vi "Rx Inline Wait.vi"(8 "error in (no error)":errorcluster, 11 "Framework in":refnum<class "Framework.lvclass">) -> (0 "error out":errorcluster, 3 "Framework out":refnum<class "Framework.lvclass">)   [LabVIEW 2021, in "DSF Core.lvlib" / "Framework.lvclass"]
uses:
  Framework.lvclass
  Framework.lvclass/Framework.ctl
  Plugin/Plugin.lvclass
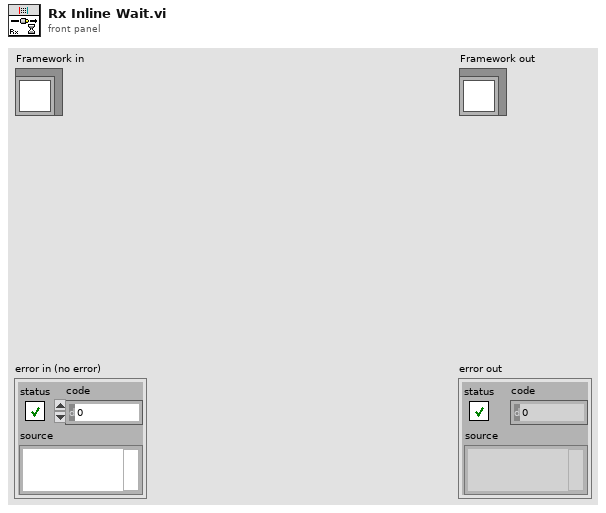
[diagram p1: front panel]
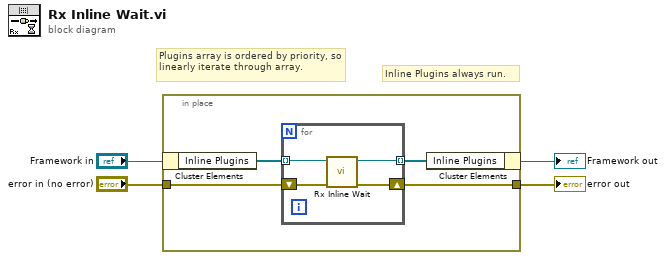
[diagram p0: block diagram]
diagram:
  # "Inline Plugins always run."
  # "Plugins array is ordered by priority, so linearly iterate through array."
  n1 = in-place {
    in-place-border: "error in (no error)" -> [w8]
    in-place-border: [w7] -> w3
    n2 = in-place-cluster #1("Framework in") -> ("Inline Plugins"=w6:refnum<class "Plugin.lvclass">[])
    n3 = for {
      tunnel: w6 -> [w9] mode=indexing
      tunnel: [w12] -> w5 mode=indexing
      shift-right: [w11] -> w7
      shift-left: w8 -> [w10]
      n4 = call "Rx Inline Wait.vi"("error in (no error)"=w10, "Plugin in"=w9) -> ("error out"=w11:errorcluster, "Plugin out"=w12:refnum<class "Plugin.lvclass">)  [unwired: 8 in]
    }
    n5 = in-place-cluster #1("Inline Plugins"=w5) -> (→"Framework out":refnum<class "Framework.lvclass">)
  }
  "error out" <- w3
